vi "Write.vi"(8 "error in (no error)":errorcluster, 9 "milliseconds to wait":u32, 10 "Write":string, 11 "Serial in":refnum<class "Serial.lvclass">) -> (0 "error out":errorcluster, 3 "Serial out":refnum<class "Serial.lvclass">)   [LabVIEW 2021, in "Communication.lvlib" / "Serial.lvclass"]
uses:
  Serial.lvclass
  Serial.lvclass/Serial.ctl
  230254f5-f17b-4599-acb5-c7c662739978.vi
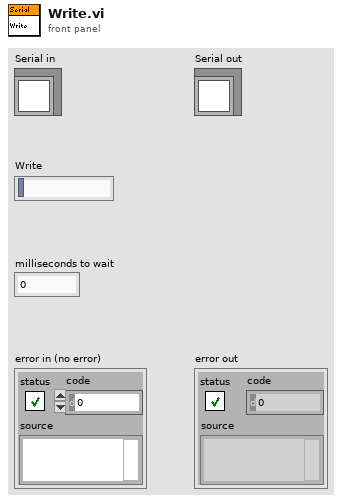
[diagram p1: front panel]
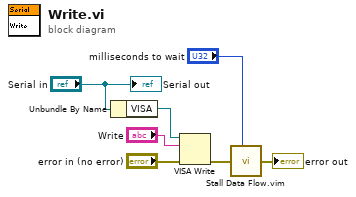
[diagram p0: block diagram]
diagram:
  n1 = Unbundle By Name("Serial in") -> ("VISA"=w7:refnum<visa-resource-name>)
  n2 = VISA Write(VISA resource name=w7, write buffer="Write", error in (no error)="error in (no error)") -> (error out=w4:errorcluster)  [unwired: 2 out]
  n3 = call "Stall Data Flow.vim"("value in"=w4, "milliseconds to wait"="milliseconds to wait") -> ("value out"=→"error out":errorcluster)  [unwired: 1 out]
  "Serial out" <- "Serial in"
